vi "ModuleClassName.vi"() -> ()   [LabVIEW 2021]
panel:
  in  "Class Name":string
  # "Error Arguments Window"
  # "Instructions: Add only Controls to this panel.\nThese controls will be used as inputs to the custom --error.vi.\nIf you don't need any arguments, leave this panel empty."
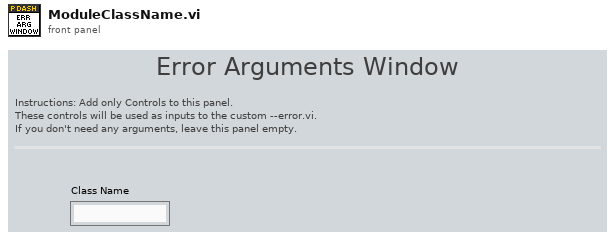
[diagram p1: front panel]
diagram:
